vi "INIT.vi"(8 "error in (no error)":errorcluster, 11 "Actor_C_MXN in":refnum<class "Actor_C_MXN.lvclass">) -> (0 "error out":errorcluster, 3 "Actor_C_MXN out":refnum<class "Actor_C_MXN.lvclass">)   [LabVIEW 2019, in "Actor_C_MXN.lvlib" / "Actor_C_MXN.lvclass"]
uses:
  Actor_C_MXN.lvclass
  Actor_C_MXN.lvclass/Actor_C_MXN.ctl
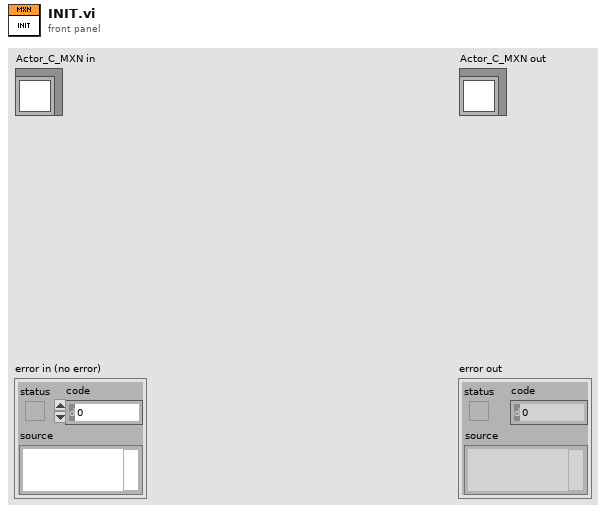
[diagram p1: front panel]
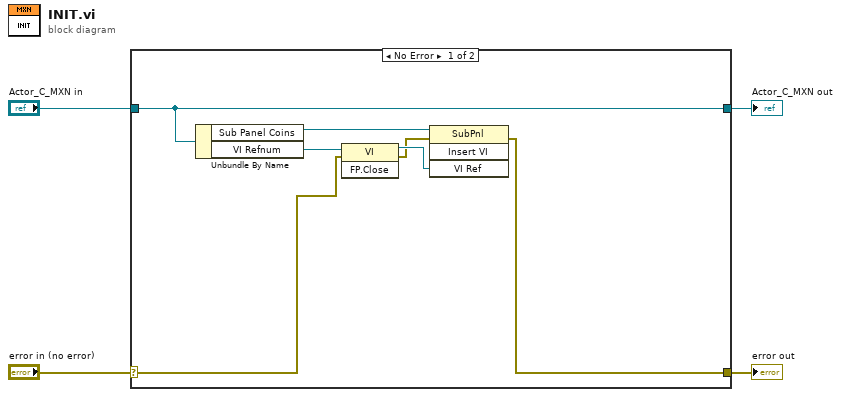
[diagram p0: block diagram]
diagram:
  n1 = case shown="No Error" "error in (no error)" {
    selector: "error in (no error)" -> [w7 w13]
    tunnel: [w6 w13] -> w3
    tunnel: [w11 w12] -> w1
    tunnel: "Actor_C_MXN in" -> [w11 w12]
    frame No Error {
      n2 = Unbundle By Name(w11) -> ("Sub Panel Coins"=w9:refnum<vi>, "VI Refnum"=w10:refnum<vi>)
      n3 = invoke class="VI" method="FP.Close"(reference=w10, error in=w7) -> (reference out=w8:refnum<vi>, error out=w5:errorcluster)  [unwired: 1 in, 1 out]
      n4 = invoke class="SubPnl" method="Insert VI"(reference=w9, error in=w5, "VI Ref"=w8) -> (error out=w6:errorcluster)  [unwired: 1 in, 3 out]
    }
    frame Error {
    }
  }
  "error out" <- w3
  "Actor_C_MXN out" <- w1
